vi "measurement perform sweeps.vi"(8 "error in (no error)":errorcluster, 11 "measurement definition":T1={"sweep parameter"=enum."angle", "sweep start"=0.0, "sweep stop"=0.0, "sweep increment"=0.0, "temperature"=0.0, "path"=path "", "magnet initial"={"magnitude"=0.0, "phi"=0.0, "theta"=0.0}, "magnet reference"={"magnitude"=0.0, "phi"=0.0, "theta"=0.0}, "const phi?"=FALSE, "delta phi (deg)"=0.5, "delta H (mT)"=0.5, "const phi init field?"=FALSE} {"magnet reference"."theta" format="%#_3g"; "magnet reference"."phi" format="%#_3g"; "magnet reference"."magnitude" format="%#_3g"; "magnet initial"."theta" format="%#_3g"; "magnet initial"."phi" format="%#_3g"; "magnet initial"."magnitude" format="%#_3g"}) -> (0 "error out":errorcluster)   [LabVIEW 2013]
uses:
  measconfig cluster.ctl
  measurement sweep parameter.ctl
  devices/magnet/magnet polar field.ctl
  measresult cluster.ctl
  measdata cluster.ctl
  devices/magnet/AMI reading polar field.ctl
  <vilib>/Analysis/1siggen.llb/Ramp Pattern by Delta.vi
  <vilib>/Analysis/NI_AALBase.lvlib
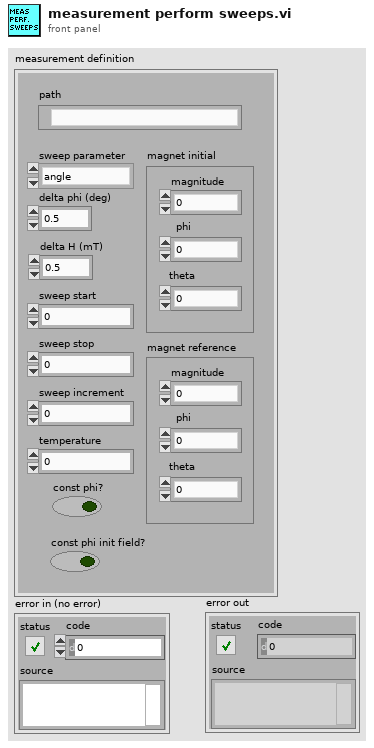
[diagram p1: front panel]
types:
  T1 = typedef "measconfig cluster.ctl" = cluster{"sweep parameter":T2, "sweep start":dbl, "sweep stop":dbl, "sweep increment":dbl, "temperature":dbl, "path":path, "magnet initial":T3, "magnet reference":T3, "const phi?":bool, "delta phi (deg)":dbl, "delta H (mT)":dbl, "const phi init field?":bool}
  T2 = typedef "measurement sweep parameter.ctl" = enum16{"angle", "magnetic field"}
  T3 = typedef "magnet polar field.ctl" = cluster{"magnitude":dbl, "phi":dbl, "theta":dbl}
  T4 = typedef "measdata cluster.ctl" = cluster{"raw data":cluster{"measurement data":dbl[][], "s-parameter":enum16{"S11", "S12", "S21", "S22"}}[], "magnetic field":T3, "reference":bool, "sweep parameter":T2, "Current Magnetic\nField\n(430 TCP reading)":T5, "current T (K)":dbl}
  T5 = typedef "AMI reading polar field.ctl" = cluster{"magnitude (T)":dbl, "phi (deg)":dbl}
  T6 = typedef "measresult cluster.ctl" = cluster{"measconfig":T1, "measdata":T4[]}
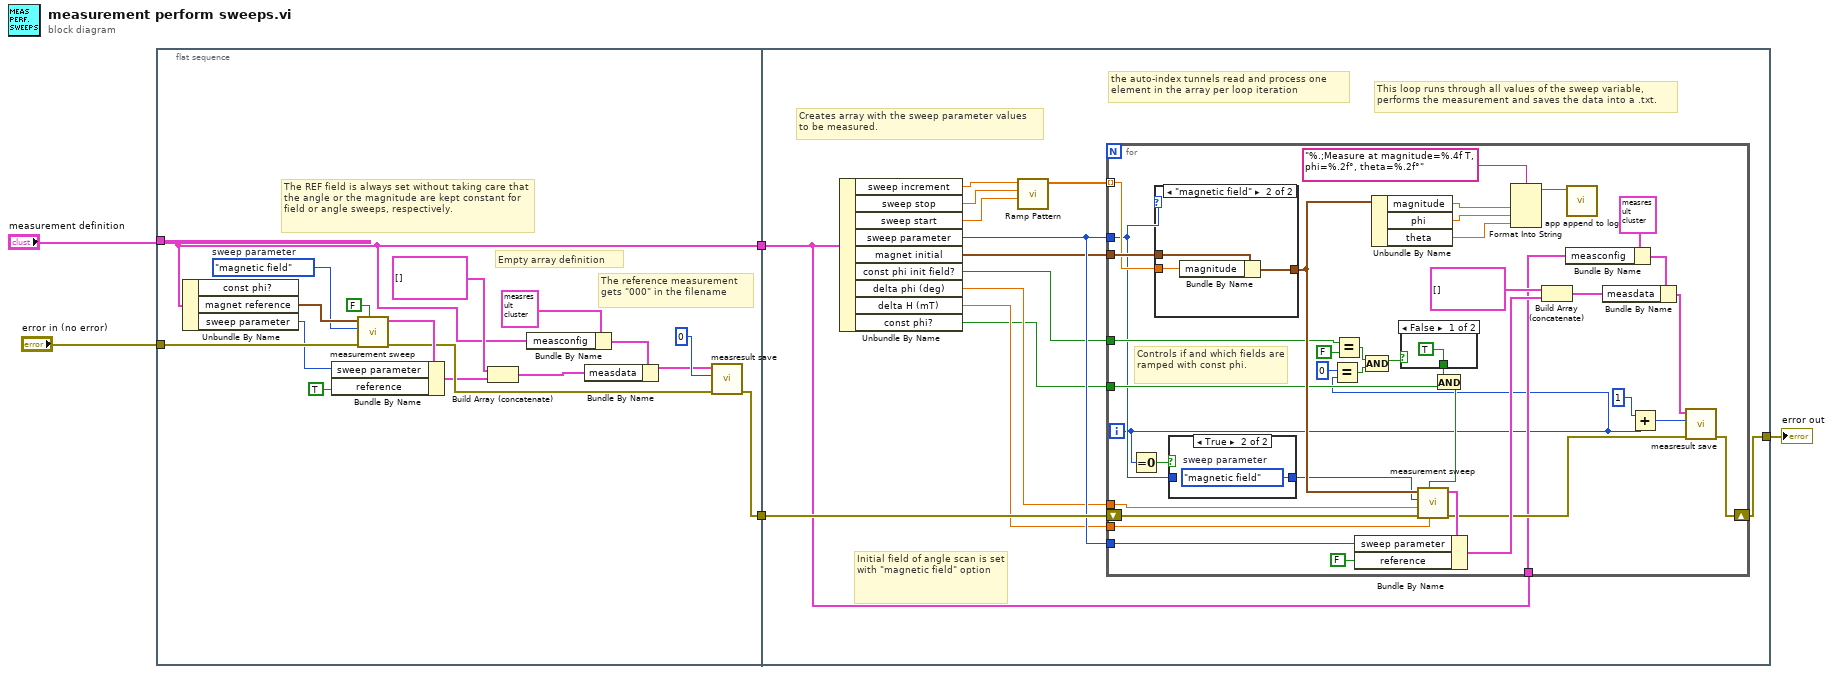
[diagram p0: block diagram]
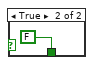
[diagram p3: hidden frame]
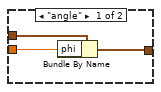
[diagram p4: hidden frame]
diagram:
  n1 = flat-sequence {
    tunnel: "error in (no error)" -> [w22]
    tunnel: "measurement definition" -> [w6]
    tunnel: [w17] -> w3
    tunnel: [w6] -> w2
    tunnel: w3 -> [w30]
    tunnel: w2 -> [w25]
    tunnel: [w31] -> w1
    frame #0 {
      w11 = measurement_sweep_parameter."magnetic field"  # sweep parameter
      # "The REF field is always set without taking care that the angle or the magnitude are kept constant for field or angle sweeps, respectively."
      # "Empty array definition"
      # "The reference measurement gets \"000\" in the filename"
      n2 = Unbundle By Name(w6) -> ("magnet reference"=w19:T3, "sweep parameter"=w13:T2)  [unwired: 1 out]
      n3 = call "measurement sweep.vi"("const phi?"=FALSE ("reference"), "error in (no error)"=w22, "sweep parameter"=w11, "magnet initial"=w19) -> ("error out"=w18:errorcluster, "measdata definition"=w20:T4)  [unwired: 6 in]
      n4 = Bundle By Name(cluster=w20, "sweep parameter"=w13, "reference"=TRUE) -> (w10:T4)
      n5 = Build Array (concatenate)(T4[] [] ("measurement result"), w10) -> (w15:T4[])
      n6 = Bundle By Name(cluster=T6 {"measconfig"={"sweep parameter"=enum."angle", "sweep start"=0.0, "sweep stop"=0.0, "sweep increment"=0.0, "temperature"=0.0, "path"=path "", "magnet initial"={"magnitude"=0.0, "phi"=0.0, "theta"=0.0}, "magnet reference"={"magnitude"=0.0, "phi"=0.0, "theta"=0.0}, "const phi?"=FALSE, "delta phi (deg)"=0.0, "delta H (mT)"=0.0, "const phi init field?"=FALSE}, "measdata"=[]} ("measresult"), "measconfig"=w6) -> (w8:T6)
      n7 = Bundle By Name(cluster=w8, "measdata"=w15) -> (w7:T6)
      n8 = call "measresult save.vi"("error in (no error)"=w18, "sort index"=0 ("index"), "measresult"=w7) -> ("error out"=w17:errorcluster)  [unwired: 8 in]
    }
    frame #1 {
      # "Initial field of angle scan is set with \"magnetic field\" option"
      # "Creates array with the sweep parameter values\nto be measured."
      # "the auto-index tunnels read and process one \nelement in the array per loop iteration"
      # "This loop runs through all values of the sweep variable,\nperforms the measurement and saves the data into a .txt."
      n9 = Unbundle By Name(w25) -> ("sweep increment"=w32:dbl, "sweep stop"=w34:dbl, "sweep start"=w33:dbl, "sweep parameter"=w29:T2, "magnet initial"=w28:T3, "const phi init field?"=w23:bool, "delta phi (deg)"=w27:dbl, "delta H (mT)"=w26:dbl, "const phi?"=w24:bool)
      n10 = call-poly <vilib>:"Ramp Pattern.vi"("start"=w33, "end"=w34, "delta"=w32) -> ("Ramp Pattern"=w35:dbl[])  [unwired: 6 in, 2 out]
      n11 = for {
        tunnel: w29 -> [w37]
        shift-right: [w58] -> w31
        shift-left: w30 -> [w73]
        tunnel: w29 -> [w70]
        tunnel: w28 -> [w72]
        tunnel: w35 -> [w62] mode=indexing
        tunnel: w24 -> [w40]
        tunnel: w27 -> [w53]
        tunnel: w26 -> [w52]
        tunnel: w25 -> [w49]
        tunnel: w23 -> [w44]
        i -> [w36]
        # "Controls if and which fields are ramped with const phi."
        n12 = Equal To 0?(x=w36) -> (x = 0?=w39:bool)
        n13 = case shown="\"magnetic field\"" w37 {
          tunnel: [w79 w82] -> w67
          tunnel: w72 -> [w80 w83]
          tunnel: w62 -> [w78 w81]
          frame "angle" {
            n14 = Bundle By Name(cluster=w80, "phi"=w78) -> (w79:T3)
          }
          frame "magnetic field" {
            n15 = Bundle By Name(cluster=w83, "magnitude"=w81) -> (w82:T3)
          }
        }
        n16 = case shown="True" w39 {
          tunnel: [w74 w75] -> w38
          tunnel: w37 -> [w74 _]
          frame False {
          }
          frame True {
            w75 = measurement_sweep_parameter."magnetic field"  # sweep parameter
          }
        }
        n17 = Equal?(x=0, y=w36) -> (x = y?=w48:bool)
        n18 = Equal?(x=w44, y=FALSE) -> (x = y?=w46:bool)
        n19 = Compound Arithmetic op=AND(w46, w48) -> (w45:bool)
        n20 = Unbundle By Name(w67) -> ("magnitude"=w66:dbl, "phi"=w65:dbl, "theta"=w64:dbl)
        n21 = case shown="False" w45 {
          tunnel: [TRUE FALSE] -> w41
          frame False {
          }
          frame True {
          }
        }
        n22 = And(x=w41, y=w40) -> (x .and. y?=w42:bool)
        n23 = call "measurement sweep.vi"("Delta H (mT)"=w52, "const phi?"=w42, "error in (no error)"=w73, "delta phi (deg)"=w53, "sweep parameter"=w38, "magnet initial"=w67) -> ("error out"=w59:errorcluster, "measdata definition"=w71:T4)  [unwired: 4 in]
        n24 = Bundle By Name(cluster=w71, "sweep parameter"=w70, "reference"=FALSE) -> (w69:T4)
        n25 = Format Into String(format string="%.;Measure at magnitude=%.4f T, phi=%.2f°, theta=%.2f°", w66, w65, w64) -> (resulting string=w63:string)  [unwired: 2 in, 1 out]
        n26 = Build Array (concatenate)(T4[] [] ("measurement result"), w69) -> (w54:T4[])
        n27 = Bundle By Name(cluster=T6 {"measconfig"={"sweep parameter"=enum."angle", "sweep start"=0.0, "sweep stop"=0.0, "sweep increment"=0.0, "temperature"=0.0, "path"=path "", "magnet initial"={"magnitude"=0.0, "phi"=0.0, "theta"=0.0}, "magnet reference"={"magnitude"=0.0, "phi"=0.0, "theta"=0.0}, "const phi?"=FALSE, "delta phi (deg)"=0.0, "delta H (mT)"=0.0, "const phi init field?"=FALSE}, "measdata"=[]} ("measresult"), "measconfig"=w49) -> (w50:T6)
        n28 = call "app append to log.vi"("log line to append"=w63) -> ()  [unwired: 11 in]
        n29 = Bundle By Name(cluster=w50, "measdata"=w54) -> (w60:T6)
        n30 = Add(x=1, y=w36) -> (x+y=w55:i32)
        n31 = call "measresult save.vi"("error in (no error)"=w59, "sort index"=w55, "measresult"=w60) -> ("error out"=w58:errorcluster)  [unwired: 8 in]
      }
    }
  }
  "error out" <- w1
